vi "Polling Control Data From PLC.vi"(8 "error in (no error)":errorcluster, 11 "TCP Network Connection in":refnum<k5>) -> (0 "error out":errorcluster, 1 "Data Read":u8[][](array[numeric]), 2 "output cluster":T1 {"Motor2ConfigData"."电流（A）" format="%.1f"; "Motor1ConfigData"."电流（A）" format="%.1f"}, 3 "TCP Network Connection out":refnum<k5>, 4 "Bool Data Valid":bool, 5 "Float Data Valid?":bool[](array[boolean]), 6 "Motor2RatingRPM":u16, 7 "Motor1RatingRPM":u16)   [LabVIEW 2018]
uses:
  Ctls/DisplayIndicator.ctl
  Ctls/MotroConfigData.ctl
  Ctls/MotorConfig.ctl
  Ctls/MagType.ctl
  Siemens S7 TCP v3_3 LV 8_5/Siemens S7 TCP v3_3 LV 8_5/S7 TCP API Library/S7 TCP.lvlib
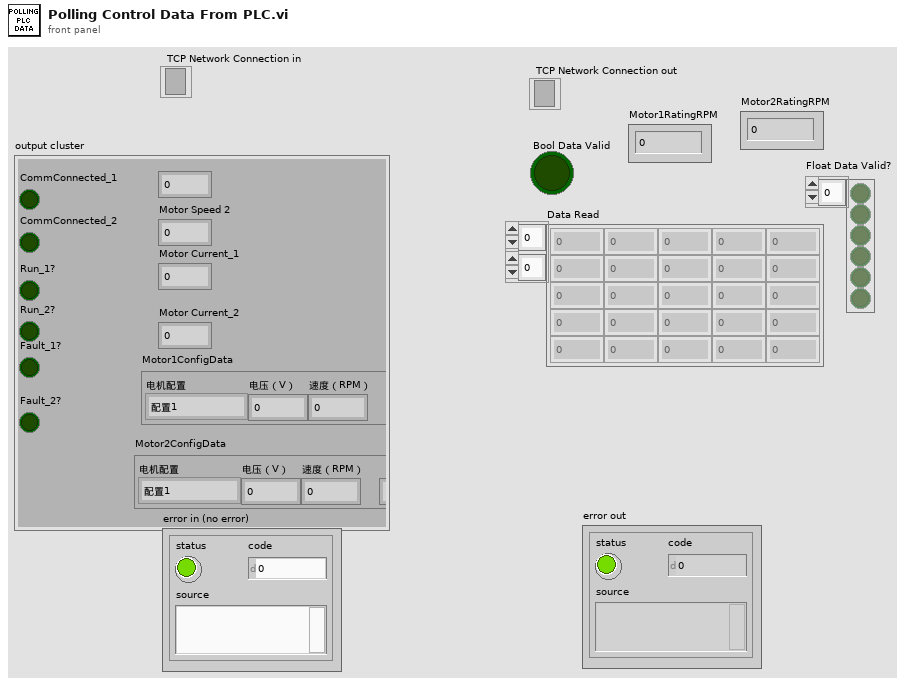
[diagram p1: front panel]
types:
  T1 = typedef "DisplayIndicator.ctl" = cluster{"CommConnected_1":bool, "Run_1?":bool, "Fault_1?":bool, "CommConnected_2":bool, "Run_2?":bool, "Fault_2?":bool, "Motor Speed 2":sgl, "Motor Speed_1":sgl, "Motor Current_1":sgl, "Motor Current_2":sgl, "Motor1ConfigData":T2, "Motor2ConfigData":T2}
  T2 = typedef "MotroConfigData.ctl" = cluster{"电机配置":T3, "电压（V）":u16, "速度（RPM）":u16, "电流（A）":u16, "励磁方式":T4}
  T3 = typedef "MotorConfig.ctl" = enum16{"配置1", "配置2", "配置3", "配置4"}
  T4 = typedef "MagType.ctl" = enum16{"永磁", "励磁"}
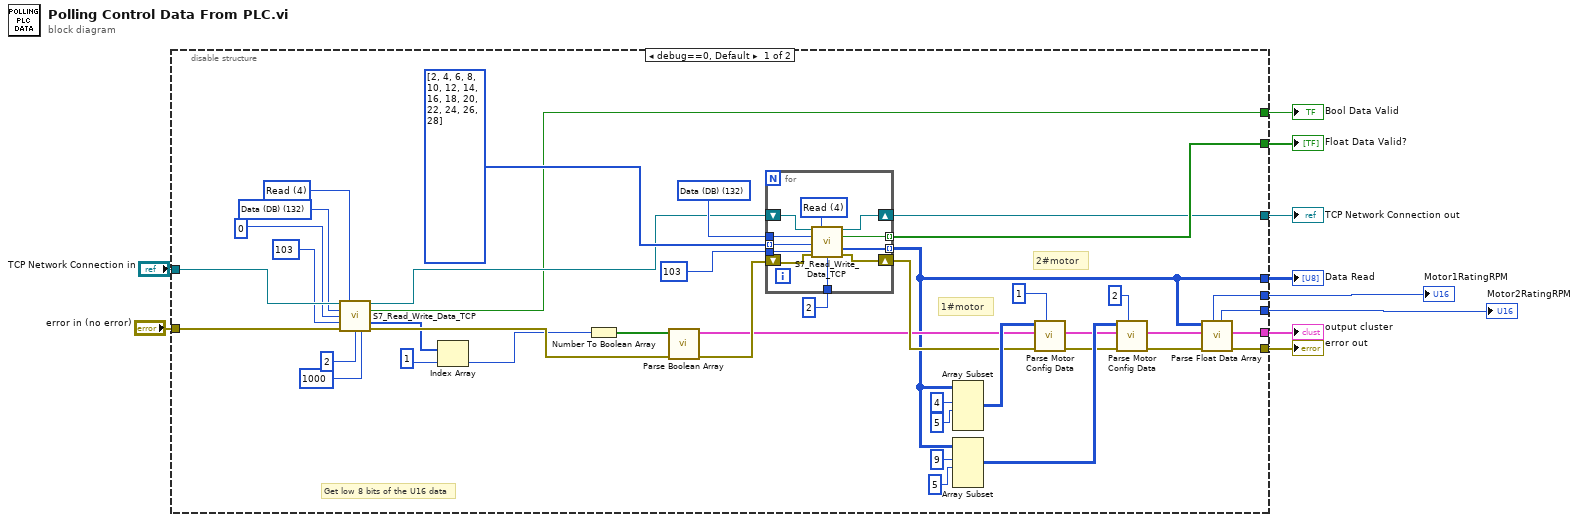
[diagram p0: block diagram]
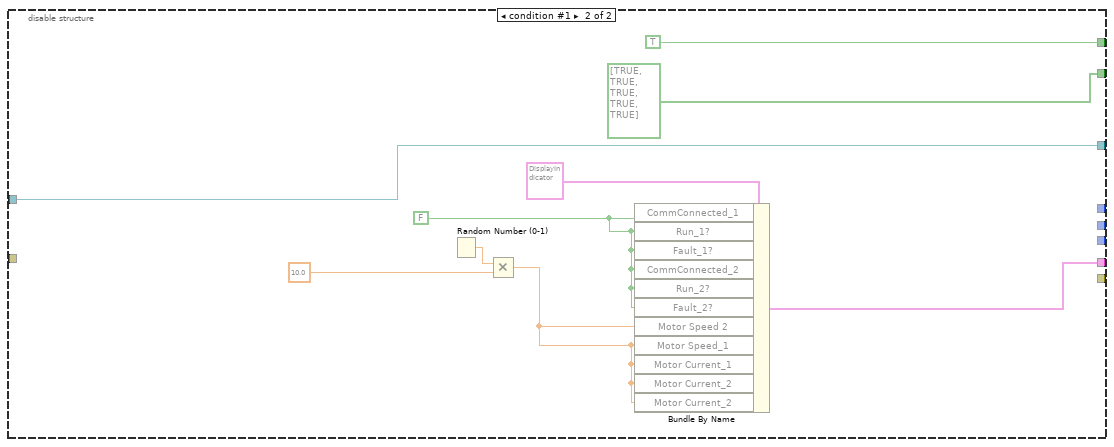
[diagram p2: hidden frame]
diagram:
  n1 = disable-structure shown="debug==0, Default" {
    disable-tunnel: [w51 w67] -> w10
    disable-tunnel: [w50 _] -> w9
    disable-tunnel: [w16 _] -> w8
    disable-tunnel: [w49 bool[] [TRUE, TRUE, TRUE, TRUE, TRUE]] -> w7
    disable-tunnel: [w44 w71] -> w6
    disable-tunnel: [w41 TRUE ("Data Valid")] -> w5
    disable-tunnel: "TCP Network Connection in" -> [w40 w71]
    disable-tunnel: "error in (no error)" -> [w39 _]
    disable-tunnel: [w13 _] -> w2
    disable-tunnel: [w12 _] -> w1
    frame condition #0 (active) {
      w33 = u8 132 items=["I/O (P)"=128, "Input (I)"=129, "Output (Q)"=130, "Bit Memory (M)"=131, "Data (DB)"=132, "Instance Data (DI)"=133, "Local Data (L)"=134, "Predecessor Local Data (VL)"=135] ("Address Areas")
      w32 = u8 4 items=["Read"=4, "Write"=5] ("Read / Write")
      w43 = u8 132 items=["I/O (P)"=128, "Input (I)"=129, "Output (Q)"=130, "Bit Memory (M)"=131, "Data (DB)"=132, "Instance Data (DI)"=133, "Local Data (L)"=134, "Predecessor Local Data (VL)"=135] ("Address Areas")
      # "2#motor"
      # "1#motor"
      # "Get low 8 bits of the U16 data"
      n2 = call "S7_Read_Write_Data_TCP.vi"("TCP Connection Ref"=w40, "Read / Write"=w32, "Address Areas"=w33, "Start Address (bytes)"=u32 0, "Data Block #"=u16 103, "error in"=w39, "Length (bytes)"=u16 2, "Timeout"=u32 1000) -> ("TCP Connection Ref Out"=w42:refnum<k5>, "Data Valid"=w41:bool, "Data Read"=w31:u8[], "error out"=w38:errorcluster)  [unwired: 2 in, 2 out]
      n3 = Index Array(array=w31, index=1) -> (element=w29:u8)
      n4 = Number To Boolean Array(number=w29) -> (Boolean array=w37:bool[])
      n5 = call "Parse Boolean Array.vi"("error in (no error)"=w38, "Bool Array Input"=w37) -> ("error out"=w47:errorcluster, "output cluster"=w19:T1)  [unwired: 8 in]
      n6 = for {
        tunnel: w43 -> [w61]
        tunnel: u16 103 ("Data Block #") -> [w58]
        tunnel: u32[] [2, 4, 6, 8, 10, 12, 14, 16, 18, 20, 22, 24, 26, 28] -> [w57] mode=indexing
        tunnel: u16 2 ("Length (bytes)") -> [w56]
        tunnel: [w55] -> w49 mode=indexing
        tunnel: [w54] -> w16 mode=indexing
        shift-right: [w52] -> w25
        shift-left: w47 -> [w53]
        shift-right: [w59] -> w44
        shift-left: w42 -> [w62]
        w60 = u8 4 items=["Read"=4, "Write"=5] ("Read / Write")
        n7 = call "S7_Read_Write_Data_TCP.vi"("TCP Connection Ref"=w62, "Read / Write"=w60, "Address Areas"=w61, "Start Address (bytes)"=w57, "Data Block #"=w58, "error in"=w53, "Length (bytes)"=w56) -> ("TCP Connection Ref Out"=w59:refnum<k5>, "Data Valid"=w55:bool, "Data Read"=w54:u8[], "error out"=w52:errorcluster)  [unwired: 3 in, 2 out]
      }
      n8 = Array Subset(array=w16, index (row)=4 ("index"), length (row)=5 ("length")) -> (w26:u8[][])  [unwired: 2 in]
      n9 = Array Subset(array=w16, index (row)=9 ("index"), length (row)=5 ("length")) -> (w22:u8[][])  [unwired: 2 in]
      n10 = call "Parse Motor Config Data.vi"("Motor NO"=u8 1, "error in (no error)"=w25, "Display"=w19, "Data Read"=w26) -> ("error out"=w21:errorcluster, "output cluster"=w18:T1)  [unwired: 6 in]
      n11 = call "Parse Motor Config Data.vi"("Motor NO"=u8 2, "error in (no error)"=w21, "Display"=w18, "Data Read"=w22) -> ("error out"=w20:errorcluster, "output cluster"=w17:T1)  [unwired: 6 in]
      n12 = call "Parse Float Data Array.vi"("error in (no error)"=w20, "Display"=w17, "Data Read"=w16) -> ("error out"=w50:errorcluster, "output cluster"=w51:T1, "Motor2RatingRPM"=w12:u16, "Motor1RatingRPM"=w13:u16)  [unwired: 5 in]
    }
    frame condition #1 {
      w66 = FALSE ("CommConnected_1")
      n13 = Random Number (0-1)() -> (number: 0 to 1=w65:dbl)
      n14 = Multiply(x=w65, y=10.0) -> (x*y=w63:dbl)
      n15 = Bundle By Name(cluster=T1 {"CommConnected_1"=FALSE, "Run_1?"=FALSE, "Fault_1?"=FALSE, "CommConnected_2"=FALSE, "Run_2?"=FALSE, "Fault_2?"=FALSE, "Motor Speed 2"=0.0, "Motor Speed_1"=0.0, "Motor Current_1"=0.0, "Motor Current_2"=0.0, "Motor1ConfigData"={"电机配置"=enum."配置1", "电压（V）"=0, "速度（RPM）"=0, "电流（A）"=0, "励磁方式"=enum."永磁"}, "Motor2ConfigData"={"电机配置"=enum."配置1", "电压（V）"=0, "速度（RPM）"=0, "电流（A）"=0, "励磁方式"=enum."永磁"}} ("output cluster"), "CommConnected_1"=w66, "Run_1?"=w66, "Fault_1?"=w66, "CommConnected_2"=w66, "Run_2?"=w66, "Fault_2?"=w66, "Motor Speed 2"=w63, "Motor Speed_1"=w63, "Motor Current_1"=w63, "Motor Current_2"=w63, "Motor Current_2"=w63) -> (w67:T1)
    }
  }
  "Bool Data Valid" <- w5
  "Float Data Valid?" <- w7
  "Data Read" <- w8
  "output cluster" <- w10
  "error out" <- w9
  "TCP Network Connection out" <- w6
  "Motor1RatingRPM" <- w2
  "Motor2RatingRPM" <- w1
